vi "MC shot tcp server.vi"(10 "notifier out":refnum<notifier>, 11 "queue out":refnum<queue>) -> ()   [LabVIEW 2020]
uses:
  tcp shot sender queue.ctl
  TCP Multiple Connections State.ctl
panel:
  out "remote address":string
  out "tcp string to send":string
  out "# of Connections":i32
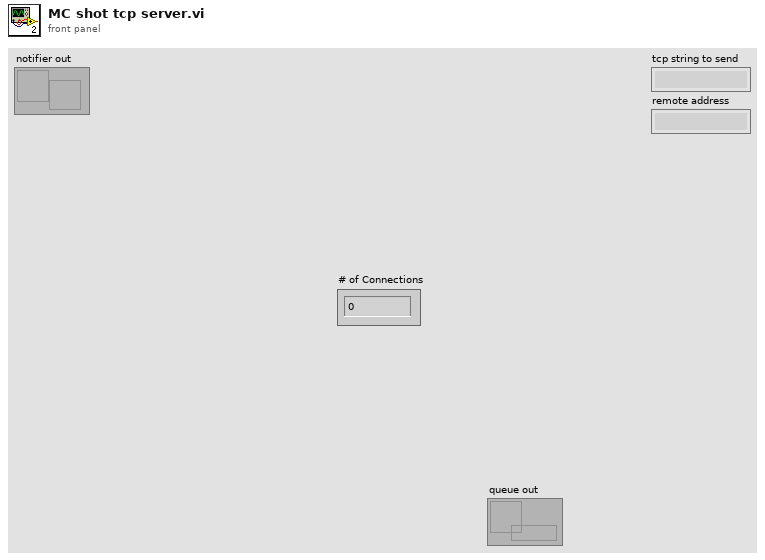
[diagram p1: front panel]
types:
  T1 = typedef "tcp shot sender queue.ctl" = cluster{"command":T2, "Number of devices":i32, "tcp string to send":string}
  T2 = typedef "TCP Multiple Connections State.ctl" = enum16{"Idle", "Initialize", "Start Scan", "Send Data", "Stop", "End Scan"}
  T3 = cluster{"Clients":refnum<k5>[], "Listener":refnum<k5>, "element":T1, "startscan tick":u32}
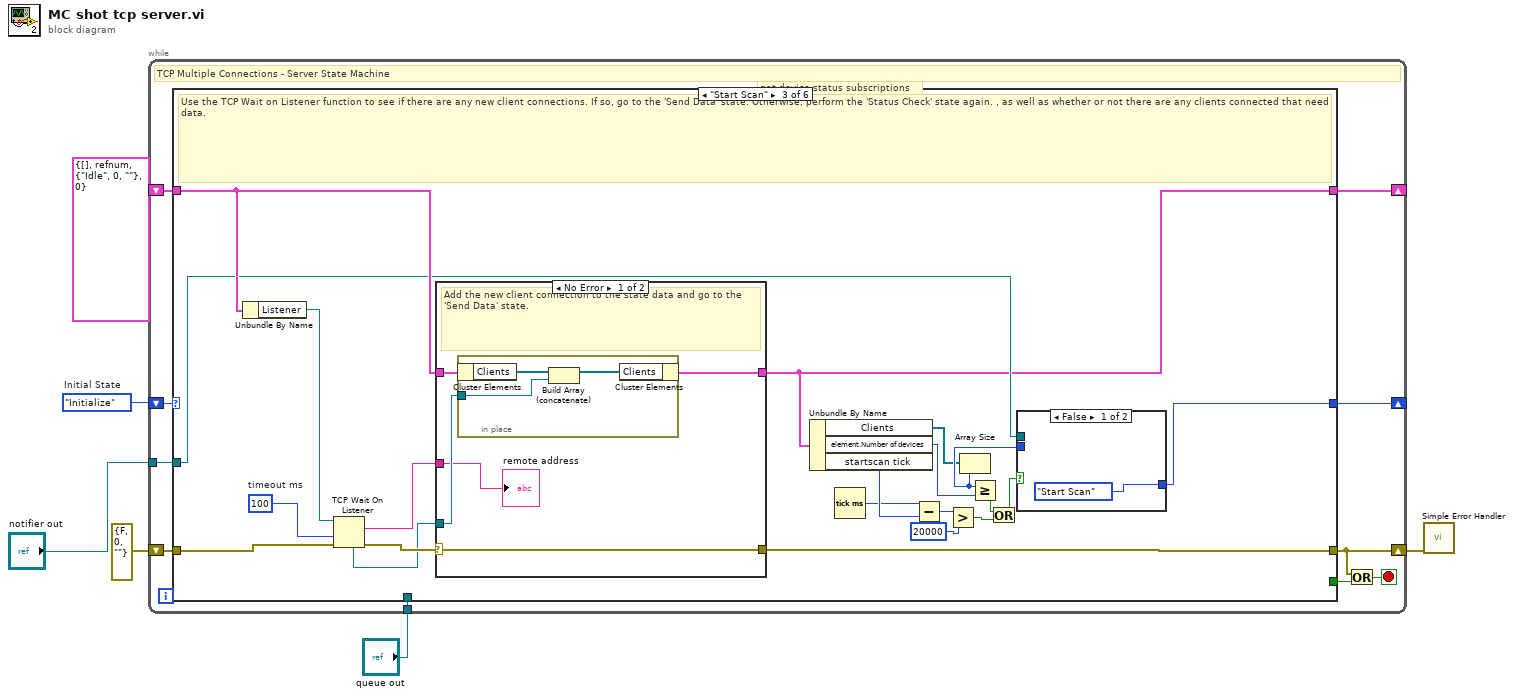
[diagram p0: block diagram]
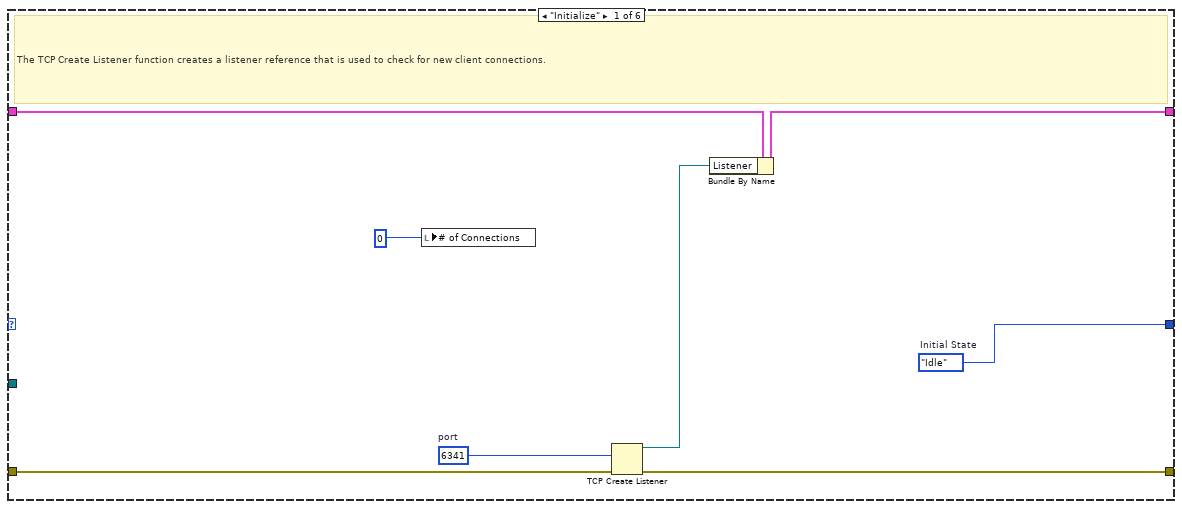
[diagram p2: hidden frame]
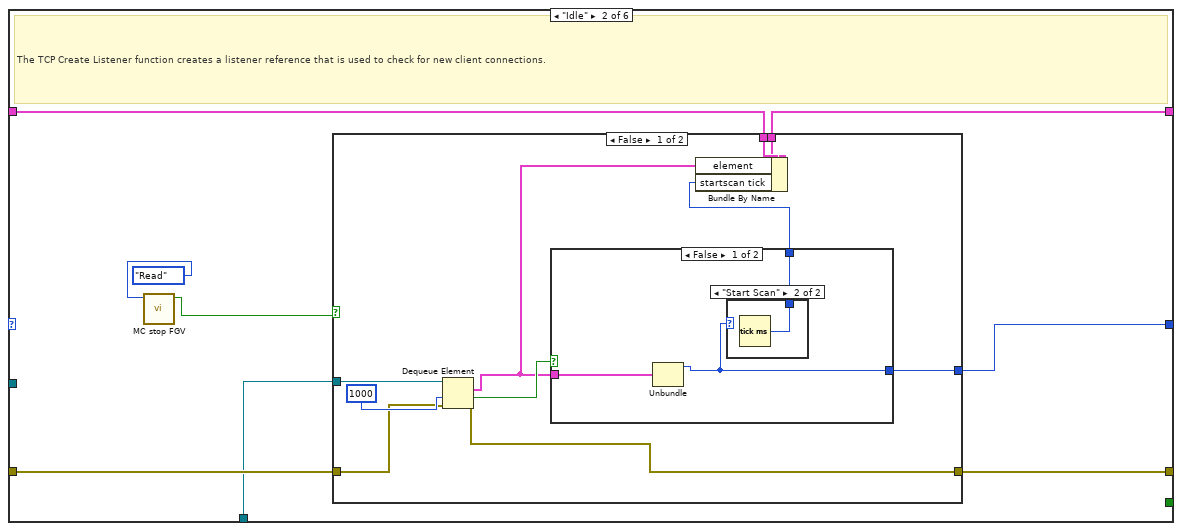
[diagram p3: hidden frame]
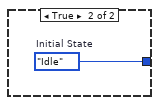
[diagram p5: hidden frame]
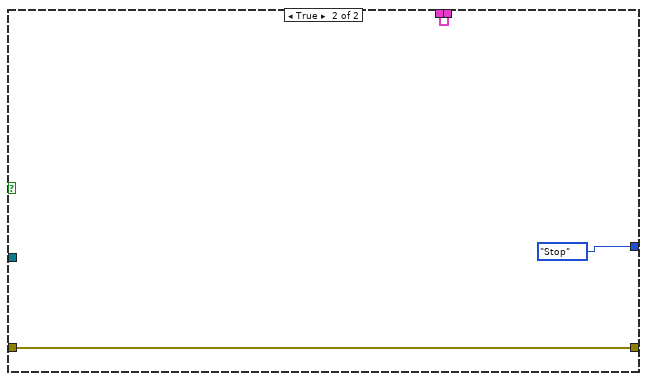
[diagram p6: hidden frame]
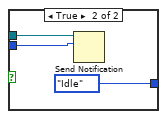
[diagram p7: hidden frame]
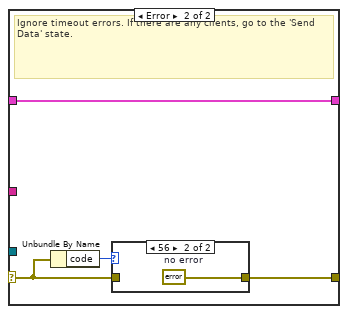
[diagram p8: hidden frame]
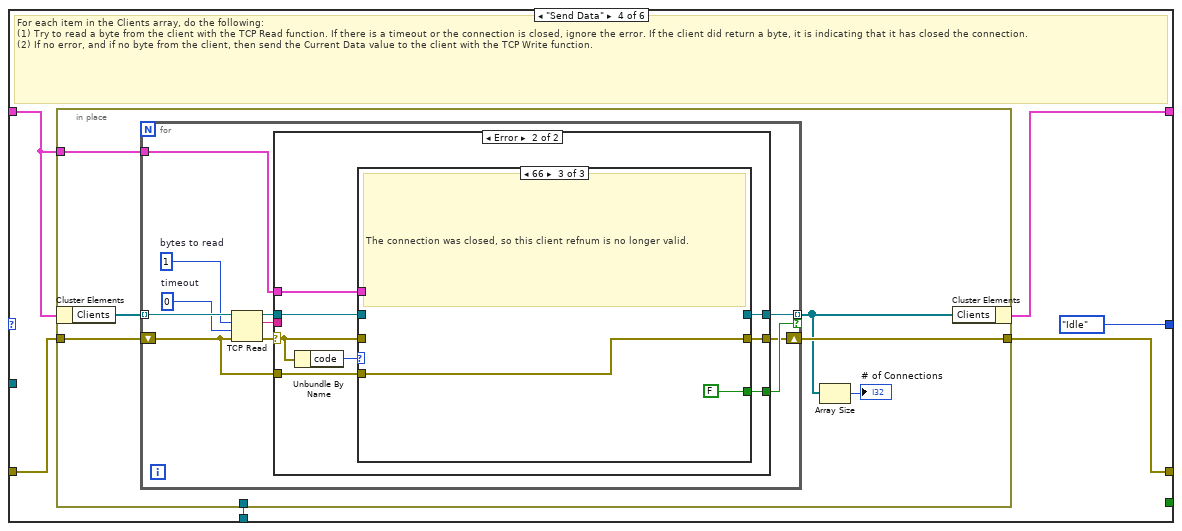
[diagram p10: hidden frame]
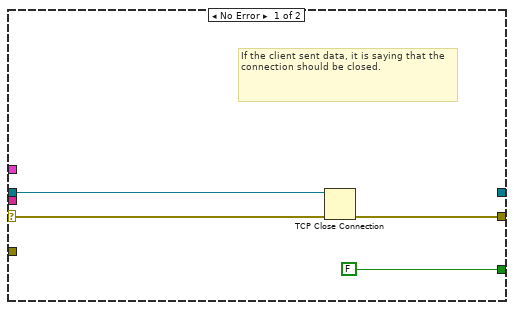
[diagram p11: hidden frame]
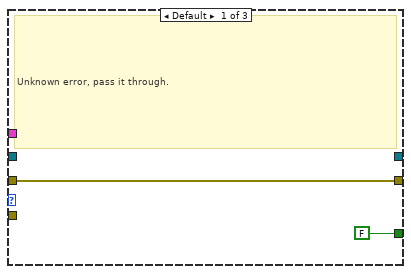
[diagram p12: hidden frame]
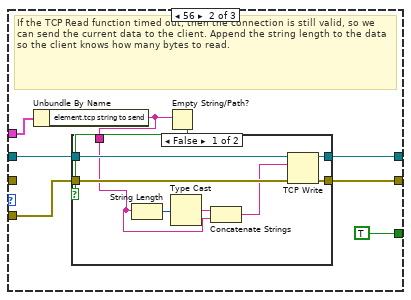
[diagram p13: hidden frame]
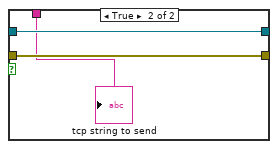
[diagram p14: hidden frame]
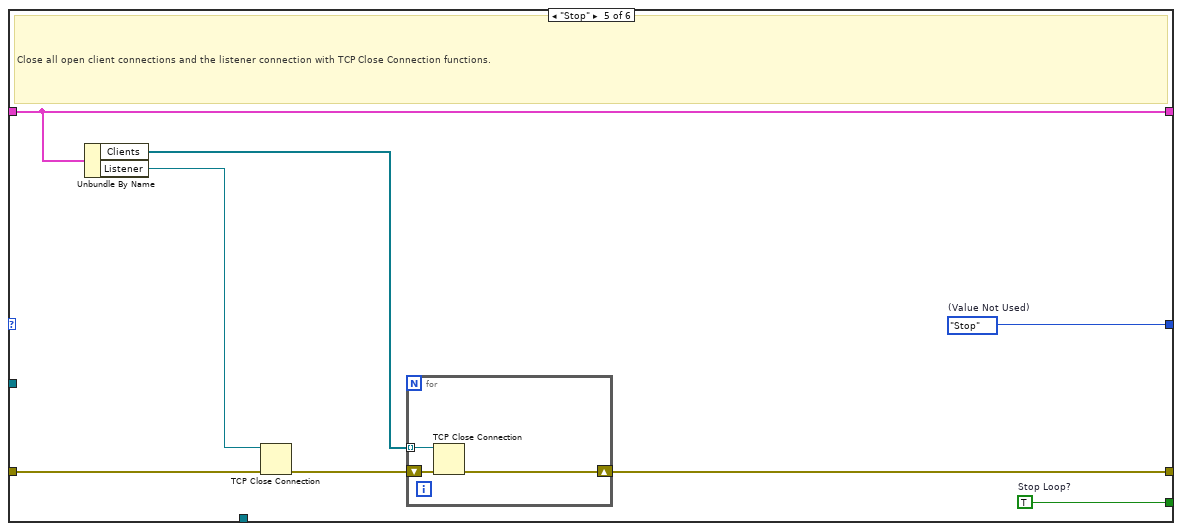
[diagram p15: hidden frame]
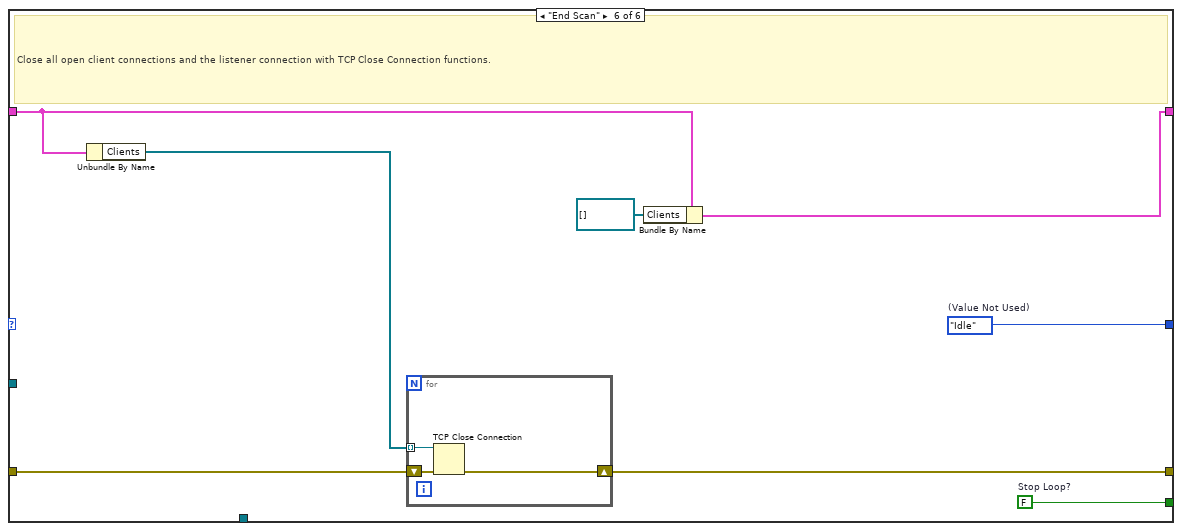
[diagram p16: hidden frame]
diagram:
  w6 = TCP_Multiple_Connections_State."Initialize"  # Initial State
  # "get device status subscriptions"
  n1 = while {
    shift-right: [w15] -> _
    shift-left: w6 -> [w16]
    shift-right: [w13] -> _
    shift-left: T3 {"Clients"=[], "Listener"=refnum, "element"={"command"=enum."Idle", "Number of devices"=0, "tcp string to send"=""}, "startscan tick"=0} ("Data") -> [w14]
    shift-right: [w9] -> w3
    shift-left: errorcluster {"status"=FALSE, "code"=0, "source"=""} ("error constant") -> [w12]
    tunnel: "queue out" -> [w8]
    tunnel: "notifier out" -> [w7]
    stop <- w10 stop-if-true
    # "TCP Multiple Connections - Server State Machine"
    n2 = case shown="\"Start Scan\"" w16 {
      tunnel: [w17 w30 w52 TCP_Multiple_Connections_State."Idle" ("States") w148 w162] -> w15
      tunnel: [_ _ _ _ w155 w166] -> w11
      tunnel: w14 -> [w22 w32 w69 w90 w154 w161]
      tunnel: [w21 w31 w51 w93 w154 w160] -> w13
      tunnel: w12 -> [w24 w29 w71 w95 w153 w165]
      tunnel: [w23 w28 w70 w94 w151 w163] -> w9
      tunnel: w8 -> [_ w27 _ w91 _ _]
      tunnel: w7 -> [_ _ w53 _ _ _]
      frame "Initialize" {
        w17 = TCP_Multiple_Connections_State."Idle"  # Initial State
        w19 = u16 6341  # port
        # "The TCP Create Listener function creates a listener reference that is used to check for new client connections."
        n3 = local write "# of Connections"(0 ("Number of Client Connections")) -> ()
        n4 = TCP Create Listener(8:w24, 10:w19) -> (0:w23:errorcluster, 3:w20:refnum<k5>)  [unwired: 4 out]
        n5 = Bundle By Name(cluster=w22, "Listener"=w20) -> (w21:T3)
      }
      frame "Idle" {
        # "The TCP Create Listener function creates a listener reference that is used to check for new client connections."
        n6 = call "MC stop FGV.vi"("Function"=enum16{"Read", "Write", "Clear"}."Read") -> ("Stop out"=w25:bool)  [unwired: 9 in, 1 out]
        n7 = case shown="False" w25 {
          tunnel: w32 -> [w42 w50]
          tunnel: [w41 w50] -> w31
          tunnel: [w40 TCP_Multiple_Connections_State."Stop" ("States")] -> w30
          tunnel: w29 -> [w38 w48]
          tunnel: [w37 w48] -> w28
          tunnel: w27 -> [w36 _]
          frame False {
            n8 = Dequeue Element(queue=w36, timeout in ms (-1)=1000, error in (no error)=w38) -> (element=w34:T1, timed out?=w35:bool, error out=w37:errorcluster)  [unwired: 1 out]
            n9 = case shown="False" w35 {
              tunnel: [w44 w47] -> w40
              tunnel: w34 -> [w45 _]
              tunnel: [w43 _] -> w33
              frame False {
                n10 = Unbundle(w45) -> ("command"=w44:T2)  [unwired: 2 out]
                n11 = case shown="\"Start Scan\"" w44 {
                  tunnel: [_ w46] -> w43
                  frame "Idle", Default {
                  }
                  frame "Start Scan" {
                    n12 = Tick Count (ms)() -> (millisecond timer value=w46:u32)
                  }
                }
              }
              frame True {
                w47 = TCP_Multiple_Connections_State."Idle"  # Initial State
              }
            }
            n13 = Bundle By Name(cluster=w42, "element"=w34, "startscan tick"=w33) -> (w41:T3)
          }
          frame True {
          }
        }
      }
      frame "Start Scan" {
        w68 = 100  # timeout ms
        # "Use the TCP Wait on Listener function to see if there are any new client connections. If so, go to the 'Send Data' state. Otherwise, perform the 'Status Check' state again. , as well as whether or not there are any clients connected that need data."
        n14 = Unbundle By Name(w69) -> ("Listener"=w65:refnum<k5>)
        n15 = TCP Wait On Listener(8:w71, 9:w68, 11:w65) -> (0:w67:errorcluster, 2:w64:string, 4:w66:refnum<k5>)  [unwired: 3 out]
        n16 = case shown="No Error" w67 {
          selector: w67 -> [w78 w87]
          tunnel: w66 -> [w79 _]
          tunnel: w69 -> [w80 w84]
          tunnel: [w77 w84] -> w51
          tunnel: [w78 w85] -> w70
          tunnel: w64 -> [w76 _]
          frame No Error {
            # "Add the new client connection to the state data and go to the 'Send Data' state."
            n17 = in-place {
              in-place-border: w79 -> [w81]
              n18 = in-place-cluster #1(w80) -> ("Clients"=w83:refnum<k5>[])
              n19 = Build Array (concatenate)(w83, w81) -> (w82:refnum<k5>[])
              n20 = in-place-cluster #1("Clients"=w82) -> (w77:T3)
            }
            "remote address" <- w76
          }
          frame Error {
            # "Ignore timeout errors. If there are any clients, go to the 'Send Data' state."
            n21 = Unbundle By Name(w87) -> ("code"=w86:i32)
            n22 = case shown="56" w86 {
              tunnel: w87 -> [w88 _]
              tunnel: [w88 w89] -> w85
              frame Default {
              }
              frame 56 {
                w89 = errorcluster {"status"=FALSE, "code"=0, "source"=""}  # no error
              }
            }
          }
        }
        n23 = Unbundle By Name(w51) -> ("Clients"=w55:refnum<k5>[], "element.Number of devices"=w56:i32, "startscan tick"=w58:u32)
        n24 = Tick Count (ms)() -> (millisecond timer value=w57:u32)
        n25 = Subtract(x=w57, y=w58) -> (x-y=w60:u32)
        n26 = Greater?(x=w60, y=u32 20000) -> (0:w61:bool)
        n27 = Array Size(array=w55) -> (size(s)=w63:i32)
        n28 = Greater Or Equal?(x=w63, y=w56) -> (x >= y?=w59:bool)
        n29 = Or(x=w59, y=w61) -> (x .or. y?=w62:bool)
        n30 = case shown="False" w62 {
          tunnel: [TCP_Multiple_Connections_State."Start Scan" ("States") TCP_Multiple_Connections_State."Idle" ("States")] -> w52
          tunnel: w53 -> [_ w74]
          tunnel: w63 -> [_ w73]
          frame False {
          }
          frame True {
            n31 = Send Notification(notification=w73, notifier=w74) -> ()  [unwired: 1 in, 2 out]
          }
        }
      }
      frame "Send Data" {
        # "For each item in the Clients array, do the following:\n(1) Try to read a byte from the client with the TCP Read function. If there is a timeout or the connection is closed, ignore the error. If the client did return a byte, it is indicating that it has closed the connection.\n(2) If no error, and if no byte from the client, then send the Current Data value to the client with the TCP Write function."
        n32 = in-place {
          in-place-border: w95 -> [w101]
          in-place-border: [w100] -> w94
          in-place-border: w91 -> [_]
          in-place-border: w90 -> [w96]
          n33 = in-place-cluster #2(w90) -> ("Clients"=w98:refnum<k5>[])
          n34 = for {
            tunnel: w98 -> [w112] mode=indexing
            shift-right: [w104] -> w100
            shift-left: w101 -> [w103]
            tunnel: [w106] -> w97 mode=indexing if=w105
            tunnel: w96 -> [w102]
            w109 = 0  # timeout
            w110 = 1  # bytes to read
            n35 = TCP Read(connection ID=w112, bytes to read=w110, error in (no error)=w103, 9:w109) -> (connection ID out=w111:refnum<k5>, data out=w107:string, error out=w108:errorcluster)  [unwired: 1 out]
            n36 = case shown="Error" w108 {
              selector: w108 -> [w115 w123]
              tunnel: w111 -> [w116 w120]
              tunnel: w107 -> [_ _]
              tunnel: [_ w118] -> w106
              tunnel: [FALSE w119] -> w105
              tunnel: [w113 w122] -> w104
              tunnel: w103 -> [_ w121]
              tunnel: w102 -> [_ w117]
              frame No Error {
                # "If the client sent data, it is saying that the connection should be closed."
                # "If the client sent data, it is saying that the connection should be closed."
                n37 = TCP Close Connection(connection ID=w116, error in (no error)=w115) -> (error out=w113:errorcluster)  [unwired: 2 out]
              }
              frame Error {
                # "Ignore connection closed and timeout errors"
                n38 = Unbundle By Name(w123) -> ("code"=w124:i32)
                n39 = case shown="66" w124 {
                  tunnel: w123 -> [w126 _ _]
                  tunnel: [w126 w134 w147] -> w122
                  tunnel: w121 -> [_ w130 w147]
                  tunnel: w120 -> [_ w133 _]
                  tunnel: [FALSE TRUE FALSE] -> w119
                  tunnel: [_ w132 _] -> w118
                  tunnel: w117 -> [_ w129 _]
                  frame Default {
                    # "Unknown error, pass it through."
                  }
                  frame 56 {
                    # "If the TCP Read function timed out, then the connection is still valid, so we can send the current data to the client. Append the string length to the data so the client knows how many bytes to read."
                    n40 = Unbundle By Name(w129) -> ("element.tcp string to send"=w128:string)
                    n41 = Empty String/Path?(string/path=w128) -> (empty?=w127:bool)
                    n42 = case shown="False" w127 {
                      tunnel: [w142 w145] -> w134
                      tunnel: w133 -> [w141 w144]
                      tunnel: [w140 w144] -> w132
                      tunnel: w130 -> [w139 w145]
                      tunnel: w128 -> [w135 w143]
                      frame False {
                        n43 = String Length(string=w135) -> (length=w137:i32)
                        n44 = Type Cast(x=w137) -> (*(type *) &x=w138:string)  [unwired: 1 in]
                        n45 = Concatenate Strings(w138, w135) -> (w136:string)
                        n46 = TCP Write(connection ID=w141, data in=w136, error in (no error)=w139) -> (connection ID out=w140:refnum<k5>, error out=w142:errorcluster)  [unwired: 2 out]
                      }
                      frame True {
                        "tcp string to send" <- w143
                      }
                    }
                  }
                  frame 66 {
                    # "The connection was closed, so this client refnum is no longer valid."
                  }
                }
              }
            }
          }
          n47 = Array Size(array=w97) -> (size(s)=→"# of Connections":i32)
          n48 = in-place-cluster #2("Clients"=w97) -> (w93:T3)
        }
      }
      frame "Stop" {
        w148 = TCP_Multiple_Connections_State."Stop"  # (Value Not Used)
        w155 = TRUE  # Stop Loop?
        # "Close all open client connections and the listener connection with TCP Close Connection functions."
        n49 = Unbundle By Name(w154) -> ("Clients"=w152:refnum<k5>[], "Listener"=w149:refnum<k5>)
        n50 = TCP Close Connection(connection ID=w149, error in (no error)=w153) -> (error out=w150:errorcluster)  [unwired: 1 in, 1 out]
        n51 = for {
          shift-right: [w157] -> w151
          shift-left: w150 -> [w158]
          tunnel: w152 -> [w156] mode=indexing
          n52 = TCP Close Connection(connection ID=w156, error in (no error)=w158) -> (error out=w157:errorcluster)  [unwired: 1 in, 1 out]
        }
      }
      frame "End Scan" {
        w162 = TCP_Multiple_Connections_State."Idle"  # (Value Not Used)
        w166 = FALSE  # Stop Loop?
        # "Close all open client connections and the listener connection with TCP Close Connection functions."
        n53 = Unbundle By Name(w161) -> ("Clients"=w164:refnum<k5>[])
        n54 = for {
          shift-right: [w168] -> w163
          shift-left: w165 -> [w169]
          tunnel: w164 -> [w167] mode=indexing
          n55 = TCP Close Connection(connection ID=w167, error in (no error)=w169) -> (error out=w168:errorcluster)  [unwired: 1 in, 1 out]
        }
        n56 = Bundle By Name(cluster=w161, "Clients"=refnum<k5>[] []) -> (w160:T3)
      }
    }
    n57 = Or(x=w9, y=w11) -> (x .or. y?=w10:bool)
  }
  n58 = call <vilib>:"Simple Error Handler.vi"("error in (no error)"=w3) -> ()  [unwired: 4 in, 5 out]
